vi "VisualInspectionAHU.vi"(8 "error in (no error)":errorcluster, 11 "TableRef":refnum<vi>) -> (0 "error out":errorcluster, 2 "VisualInspectionResult":bool)   [LabVIEW 2017]
panel:
  in  "14.3":dbl
  in  "11":dbl
  in  "15.1":dbl
  in  "14.2":dbl
  in  "14.1":dbl
  in  "13.2":dbl
  in  "13.1":dbl
  in  "12.1":dbl
  in  "10.4":dbl
  in  "10.3":dbl
  in  "10.2":dbl
  in  "10.1":dbl
  in  "9.1":dbl
  in  "16":bool
  in  "8.2":bool
  in  "8.1":bool
  in  "Cancel Button":bool
  in  "OK Button":bool
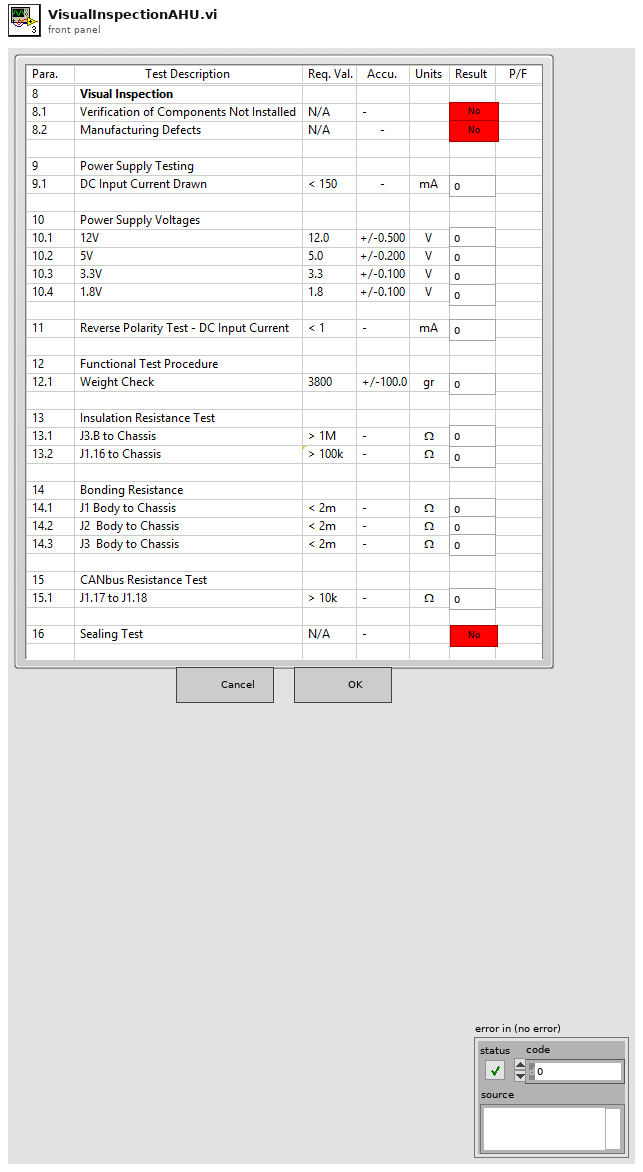
[diagram p1: front panel]
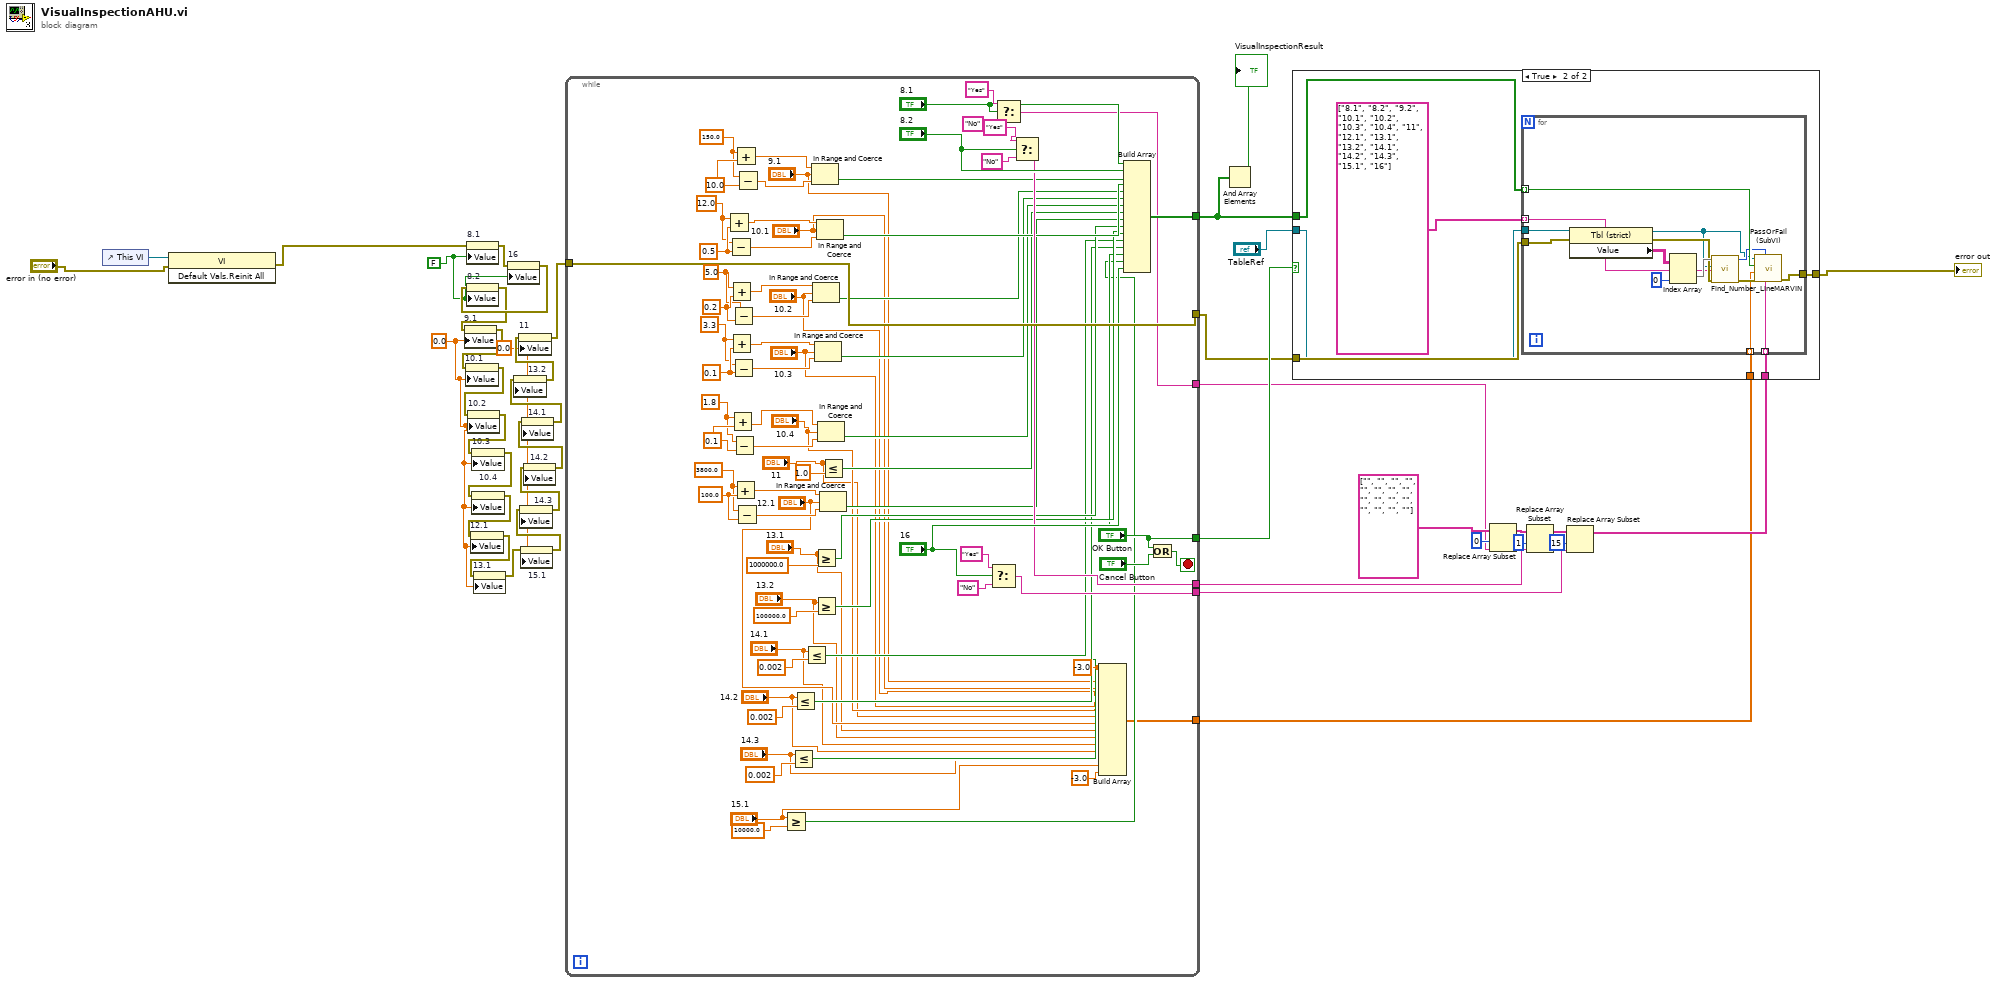
[diagram p0: block diagram]
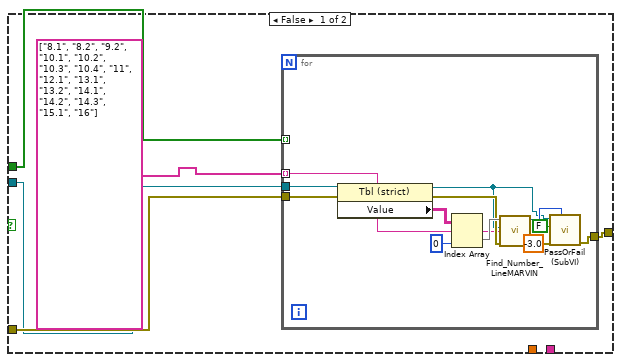
[diagram p2: hidden frame]
diagram:
  w1 = FALSE
  w2 = 0.0 ("11")
  w3 = 0.0 ("11")
  n1 = control-ref of="This VI"() -> (w36:refnum<vi>)
  n2 = invoke class="VI" method="Default Vals.Reinit All"(reference=w36, error in="error in (no error)") -> (error out=w20:errorcluster)  [unwired: 1 in, 2 out]
  n3 = property on="8.1" class="Bool (strict)"(error in=w20, "Value"=w1) -> (error out=w19:errorcluster)  [unwired: 1 in, 1 out]
  n4 = property on="16" class="Bool (strict)"(error in=w19, "Value"=w1) -> (error out=w18:errorcluster)  [unwired: 1 in, 1 out]
  n5 = property on="8.2" class="Bool (strict)"(error in=w18, "Value"=w1) -> (error out=w17:errorcluster)  [unwired: 1 in, 1 out]
  n6 = property on="9.1" class="DigNum (strict)"(error in=w17, "Value"=w2) -> (error out=w16:errorcluster)  [unwired: 1 in, 1 out]
  n7 = property on="10.1" class="DigNum (strict)"(error in=w16, "Value"=w2) -> (error out=w15:errorcluster)  [unwired: 1 in, 1 out]
  n8 = property on="10.2" class="DigNum (strict)"(error in=w15, "Value"=w2) -> (error out=w14:errorcluster)  [unwired: 1 in, 1 out]
  n9 = property on="10.3" class="DigNum (strict)"(error in=w14, "Value"=w2) -> (error out=w13:errorcluster)  [unwired: 1 in, 1 out]
  n10 = property on="10.4" class="DigNum (strict)"(error in=w13, "Value"=w2) -> (error out=w12:errorcluster)  [unwired: 1 in, 1 out]
  n11 = property on="12.1" class="DigNum (strict)"(error in=w12, "Value"=w2) -> (error out=w11:errorcluster)  [unwired: 1 in, 1 out]
  n12 = property on="13.1" class="DigNum (strict)"(error in=w11, "Value"=w2) -> (error out=w10:errorcluster)  [unwired: 1 in, 1 out]
  n13 = property on="15.1" class="DigNum (strict)"(error in=w10, "Value"=w3) -> (error out=w9:errorcluster)  [unwired: 1 in, 1 out]
  n14 = property on="14.3" class="DigNum (strict)"(error in=w9, "Value"=w3) -> (error out=w8:errorcluster)  [unwired: 1 in, 1 out]
  n15 = property on="14.2" class="DigNum (strict)"(error in=w8, "Value"=w3) -> (error out=w7:errorcluster)  [unwired: 1 in, 1 out]
  n16 = property on="14.1" class="DigNum (strict)"(error in=w7, "Value"=w3) -> (error out=w6:errorcluster)  [unwired: 1 in, 1 out]
  n17 = property on="13.2" class="DigNum (strict)"(error in=w6, "Value"=w3) -> (error out=w5:errorcluster)  [unwired: 1 in, 1 out]
  n18 = property on="11" class="DigNum (strict)"(error in=w5, "Value"=w3) -> (error out=w4:errorcluster)  [unwired: 1 in, 1 out]
  n19 = while {
    tunnel: w4 -> [w112]
    tunnel: [w114] -> w33
    tunnel: ["OK Button"] -> w39
    tunnel: [w112] -> w38
    tunnel: [w72] -> w25
    tunnel: [w71] -> w24
    tunnel: [w70] -> w23
    tunnel: [w40] -> w21
    stop <- w115 stop-if-true
    w55 = -3.0 ("element")
    w91 = 0.5 ("y")
    w93 = 0.2 ("y")
    w95 = 0.1 ("y")
    w97 = 0.1 ("y")
    w99 = 100.0 ("y")
    w89 = 10.0 ("y")
    w98 = 3800.0 ("y")
    w96 = 1.8 ("y")
    w94 = 3.3 ("y")
    w92 = 5.0 ("y")
    w90 = 12.0 ("y")
    w88 = 150.0 ("y")
    n20 = Add(x=w90, y=w91) -> (x+y=w102:dbl)
    n21 = Subtract(x=w90, y=w91) -> (x-y=w103:dbl)
    n22 = Add(x=w92, y=w93) -> (x+y=w104:dbl)
    n23 = Add(x=w94, y=w95) -> (x+y=w106:dbl)
    n24 = Add(x=w96, y=w97) -> (x+y=w108:dbl)
    n25 = Subtract(x=w92, y=w93) -> (x-y=w105:dbl)
    n26 = Subtract(x=w94, y=w95) -> (x-y=w107:dbl)
    n27 = Subtract(x=w96, y=w97) -> (x-y=w109:dbl)
    n28 = Add(x=w98, y=w99) -> (x+y=w110:dbl)
    n29 = Add(x=w88, y=w89) -> (x+y=w100:dbl)
    n30 = Subtract(x=w98, y=w99) -> (x-y=w111:dbl)
    n31 = Subtract(x=w88, y=w89) -> (x-y=w101:dbl)
    n32 = Greater Or Equal?(x="15.1", y=10000.0) -> (x >= y?=w56:bool)
    n33 = Less Or Equal?(x="14.3", y=0.002) -> (x <= y?=w57:bool)
    n34 = Less Or Equal?(x="14.2", y=0.002) -> (x <= y?=w58:bool)
    n35 = Less Or Equal?(x="14.1", y=0.002) -> (x <= y?=w59:bool)
    n36 = In Range and Coerce(upper limit=w100, x="9.1", lower limit=w101) -> (In Range?=w68:bool)  [unwired: 1 out]
    n37 = In Range and Coerce(upper limit=w104, x="10.2", lower limit=w105) -> (In Range?=w66:bool)  [unwired: 1 out]
    n38 = Greater Or Equal?(x="13.1", y=1000000.0) -> (x >= y?=w61:bool)
    n39 = Greater Or Equal?(x="13.2", y=100000.0) -> (x >= y?=w60:bool)
    n40 = In Range and Coerce(upper limit=w106, x="10.3", lower limit=w107) -> (In Range?=w65:bool)  [unwired: 1 out]
    n41 = In Range and Coerce(upper limit=w102, x="10.1", lower limit=w103) -> (In Range?=w67:bool)  [unwired: 1 out]
    n42 = In Range and Coerce(upper limit=w108, x="10.4", lower limit=w109) -> (In Range?=w64:bool)  [unwired: 1 out]
    n43 = Less Or Equal?(x="11", y=1.0) -> (x <= y?=w63:bool)
    n44 = In Range and Coerce(upper limit=w110, x="12.1", lower limit=w111) -> (In Range?=w62:bool)  [unwired: 1 out]
    n45 = Select(t="Yes", s="16", f="No") -> (s? t:f=w70:string)
    n46 = Select(t="Yes", s="8.1", f="No") -> (s? t:f=w72:string)
    n47 = Select(t="Yes", s="8.2", f="No") -> (s? t:f=w71:string)
    n48 = Build Array(w55, w55, "9.1", "10.1", "10.2", "10.3", "10.4", "11", "12.1", "13.1", "13.2", "14.1", "14.2", "14.3", "15.1", -3.0 ("element")) -> (w40:dbl[])
    n49 = Build Array("8.1", "8.2", w68, w67, w66, w65, w64, w63, w62, w61, w60, w59, w58, w57, w56, "16") -> (w114:bool[])
    n50 = Or(x="OK Button", y="Cancel Button") -> (x .or. y?=w115:bool)
  }
  n51 = And Array Elements(Boolean array=w33) -> (logical AND=→"VisualInspectionResult":bool)
  n52 = Replace Array Subset(array=string[] ["", "", "", "", "", "", "", "", "", "", "", "", "", "", "", ""], new element=w25, index=0) -> (w30:string[])
  n53 = Replace Array Subset(array=w30, new element=w24, index=1) -> (w29:string[])
  n54 = Replace Array Subset(array=w29, new element=w23, index=15) -> (w22:string[])
  n55 = case shown="True" w39 {
    tunnel: w33 -> [w121 w141]
    tunnel: w38 -> [w120 w140]
    tunnel: [w119 w139] -> w34
    tunnel: "TableRef" -> [w118 w138]
    tunnel: w22 -> [_ w136]
    tunnel: w21 -> [_ w135]
    frame False {
      n56 = for {
        tunnel: string[] ["8.1", "8.2", "9.2", "10.1", "10.2", "10.3", "10.4", "11", "12.1", "13.1", "13.2", "14.1", "14.2", "14.3", "15.1", "16"] ("Array 3") -> [w130] mode=indexing
        tunnel: w121 -> [_] mode=indexing
        tunnel: w120 -> [w127]
        tunnel: [w126] -> w119
        tunnel: w118 -> [w125]
        n57 = property class="Tbl (strict)"(reference=w125, error in=w127) -> (reference out=w122:refnum<vi>, error out=w131:errorcluster, "Value"=w134:string[][])
        n58 = Index Array(array=w134, index (col)=0 ("disabled index (col)")) -> (element=w132:string[])  [unwired: 1 in]
        n59 = call "Find_Number_LineMARVIN.vi"("Test Paragraph"=w130, "error in"=w131, "TableIn"=w122, "Row Headers[]"=w132) -> ("error out"=w129:errorcluster, "Line number"=w128:i32)  [unwired: 1 in, 2 out]
        n60 = call "PassOrFail (SubVI).vi"("index (row)"=w128, "error in (no error)"=w129, "Data in"=-3.0, "Pass?Fail"=FALSE ("Boolean"), "Table in"=w122) -> ("error out"=w126:errorcluster)  [unwired: 6 in]
      }
    }
    frame True {
      n61 = for {
        tunnel: string[] ["8.1", "8.2", "9.2", "10.1", "10.2", "10.3", "10.4", "11", "12.1", "13.1", "13.2", "14.1", "14.2", "14.3", "15.1", "16"] ("Array 3") -> [w151] mode=indexing
        tunnel: w141 -> [w149] mode=indexing
        tunnel: w140 -> [w147]
        tunnel: [w146] -> w139
        tunnel: w138 -> [w145]
        tunnel: w136 -> [w143] mode=indexing
        tunnel: w135 -> [w142] mode=indexing
        n62 = property class="Tbl (strict)"(reference=w145, error in=w147) -> (reference out=w144:refnum<vi>, error out=w152:errorcluster, "Value"=w155:string[][])
        n63 = Index Array(array=w155, index (col)=0 ("disabled index (col)")) -> (element=w153:string[])  [unwired: 1 in]
        n64 = call "Find_Number_LineMARVIN.vi"("Test Paragraph"=w151, "error in"=w152, "TableIn"=w144, "Row Headers[]"=w153) -> ("error out"=w150:errorcluster, "Line number"=w148:i32)  [unwired: 1 in, 2 out]
        n65 = call "PassOrFail (SubVI).vi"("String Res"=w143, "index (row)"=w148, "error in (no error)"=w150, "Data in"=w142, "Pass?Fail"=w149, "Table in"=w144) -> ("error out"=w146:errorcluster)  [unwired: 5 in]
      }
    }
  }
  "error out" <- w34
